vi "OpenMainDB.vi"() -> (0 "头信息":string)   [LabVIEW 2014]
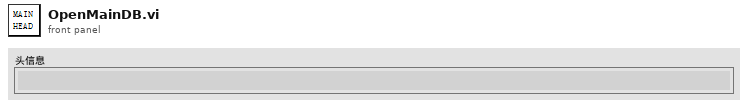
[diagram p1: front panel]
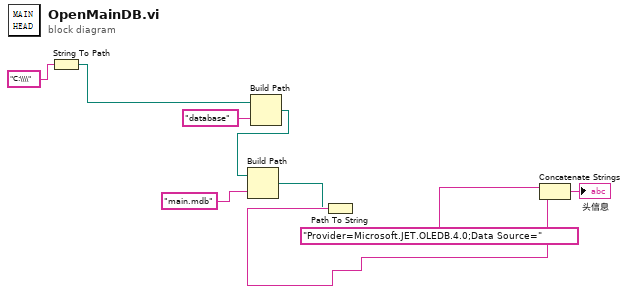
[diagram p0: block diagram]
diagram:
  n1 = String To Path(string="C:\\\\") -> (path=w1:path)
  n2 = Build Path(base path=w1, name or relative path="database" ("名称或相对路径")) -> (appended path=w5:path)
  n3 = Build Path(base path=w5, name or relative path="main.mdb" ("名称或相对路径")) -> (appended path=w4:path)
  n4 = Path To String(path=w4) -> (string=w9:string)
  n5 = Concatenate Strings("Provider=Microsoft.JET.OLEDB.4.0;Data Source=", w9) -> (→"头信息":string)
